vi "Read Temp Image.vi"(8 "error in (no error)":errorcluster, 11 "CS250-CameraHardwareClass in":refnum<class "CS250-CameraHardwareClass.lvclass">) -> (0 "error out":errorcluster, 2 "Image":T1, 3 "CS250-CameraHardwareClass out":refnum<class "CS250-CameraHardwareClass.lvclass">)   [LabVIEW 2013, in "CS250-CameraHardwareClass.lvclass"]
uses:
  CS250-CameraHardwareClass.lvclass
  <vilib>/vision/Image Controls.llb/IMAQ Image.ctl
  CS250-CameraHardwareClass.lvclass/CS250-CameraHardwareClass.ctl
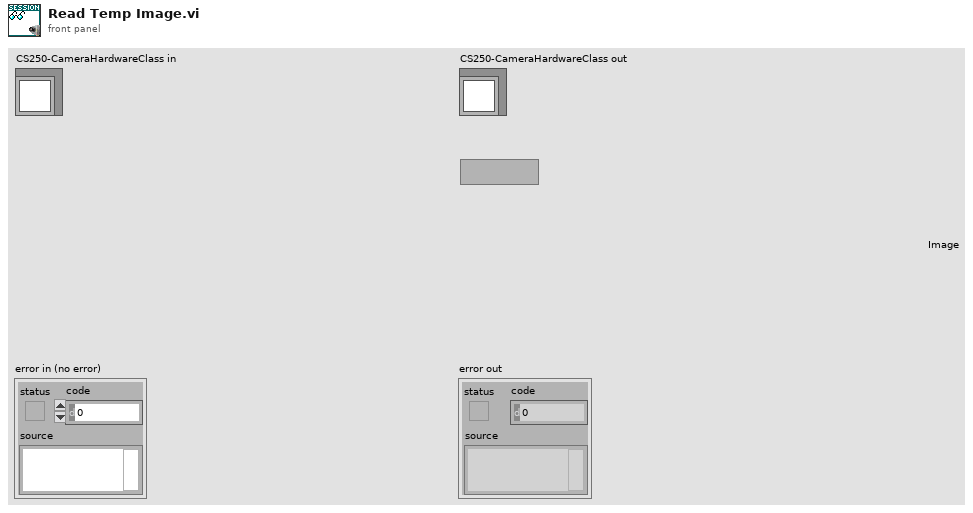
[diagram p1: front panel]
types:
  T1 = typedef "IMAQ Image.ctl" = refnum<image>
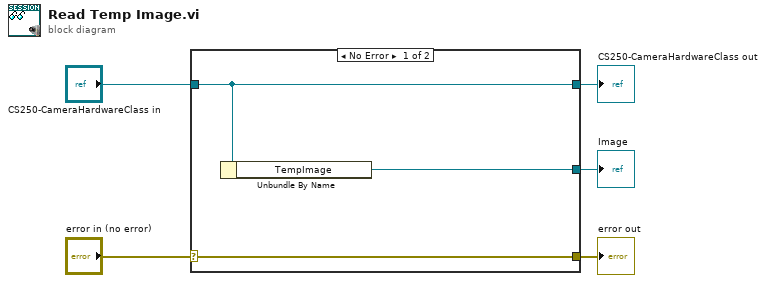
[diagram p0: block diagram]
diagram:
  n1 = case shown="No Error" "error in (no error)" {
    selector: "error in (no error)" -> [w8 w9]
    tunnel: [w8 w9] -> w4
    tunnel: [w7 w10] -> w2
    tunnel: "CS250-CameraHardwareClass in" -> [w7 w10]
    tunnel: [w6 _] -> w1
    frame No Error {
      n2 = Unbundle By Name(w7) -> ("TempImage"=w6:T1)
    }
    frame Error {
    }
  }
  "error out" <- w4
  "CS250-CameraHardwareClass out" <- w2
  "Image" <- w1
